vi "sub_EasyIsel.vi"(0 "x-Position":dbl, 1 "y-Position":dbl, 2 "z-Position":dbl, 3 "Velocity (x)":dbl=2000.0, 4 "Velocity (y)":dbl=500.0, 5 "Velocity (z)":dbl=4000.0, 6 "VISA resource name":refnum<visa-resource-name>="COM4", 8 "Mode":enum16{"Position", "Move", "Stop", "Home"}(ring), 9 "Steps/mm (y)":dbl=157.0, 11 "Steps/mm (z)":dbl=157.0) -> (14 "x-Position":dbl=6428.828025477707, 15 "y-Position":dbl, 16 "z-Position":dbl, 17 "Errorcode":string)   [LabVIEW 2014]
uses:
  <vilib>/Instr/_visa.llb/VISA Configure Serial Port (Instr).vi
panel:
  in  "Steps/mm (x)":dbl=157.0
  # "Set Steps/mm (x) to 157! (Markus)"
  # "Set Steps/mm (z) to 157! (Markus)"
  # "Description:\n\nFour different modes: Move, Position, Home, Stop\n\nMove: Move to position (absolute)\n\nPosition: Get position (x, y, z)\n\nHome: Set home\n\nStop: Stops movement and writes position (but resets controller -> new home)"
  # "Manuel Weiss, 13.08.2015"
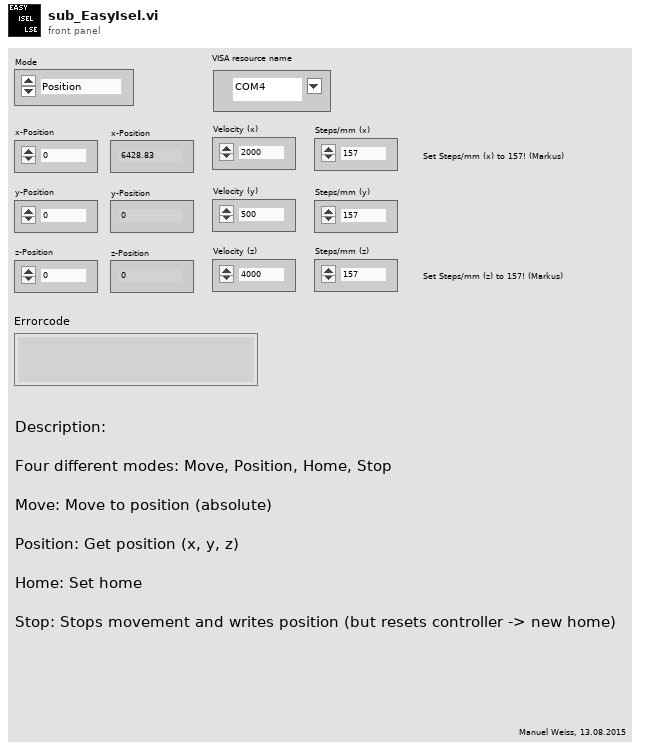
[diagram p1: front panel]
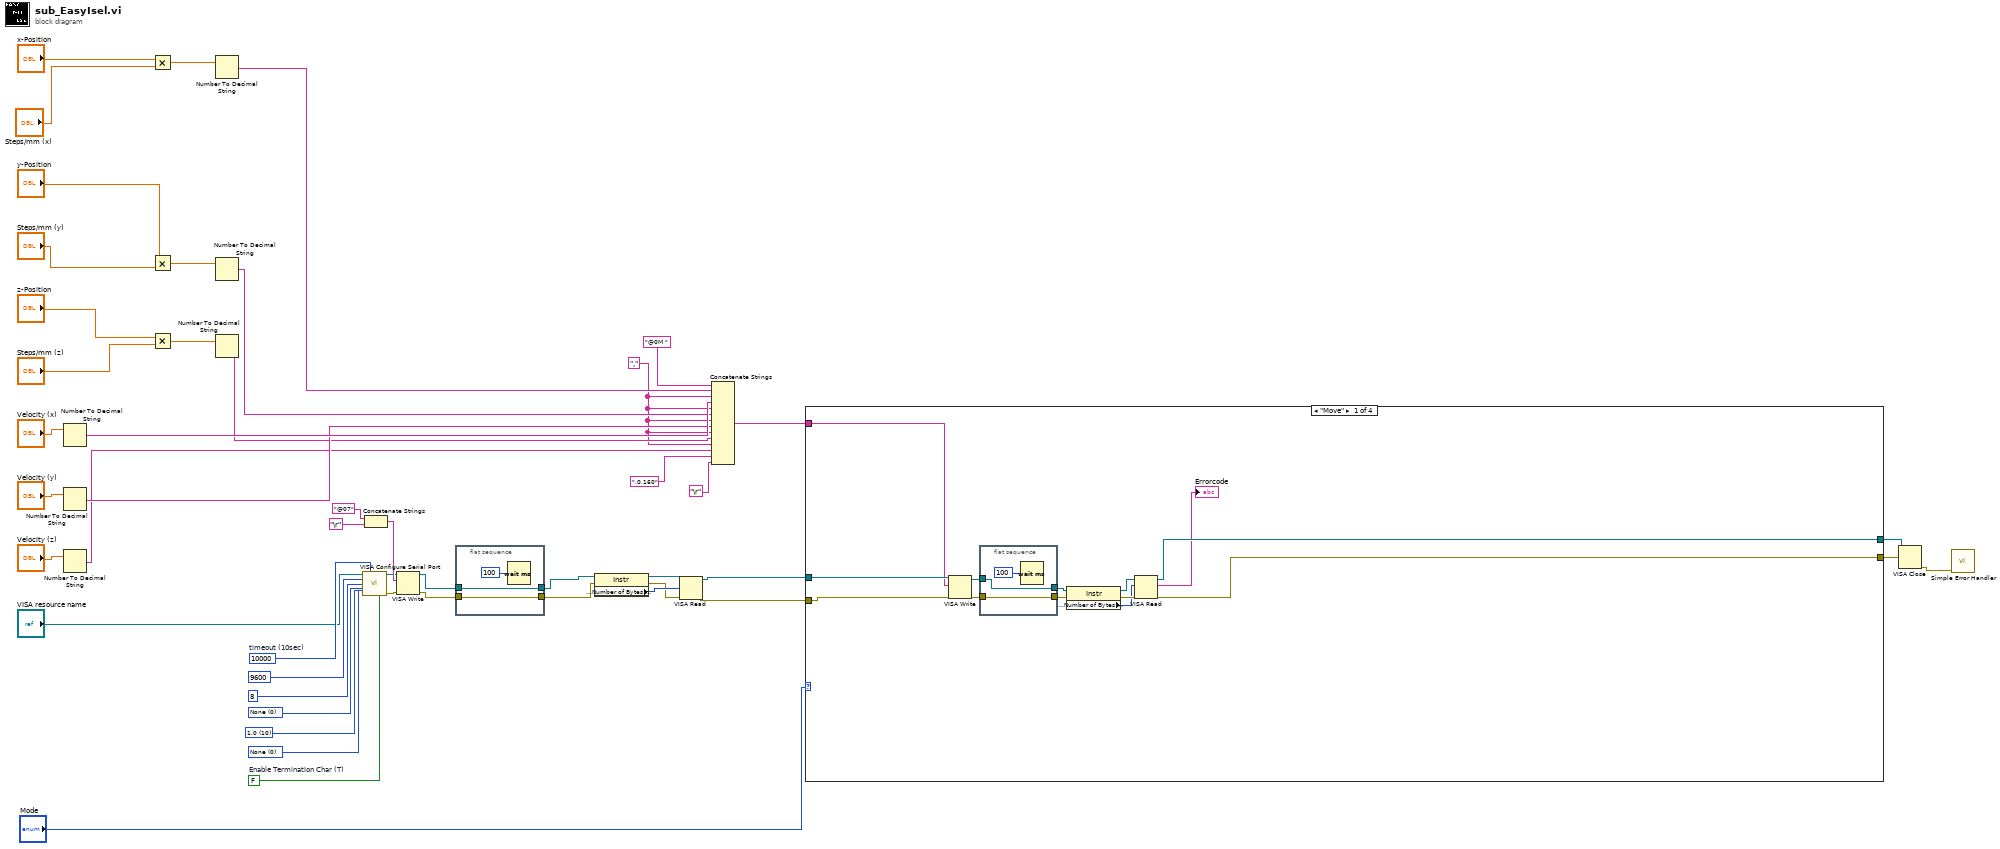
[diagram p0: block diagram]
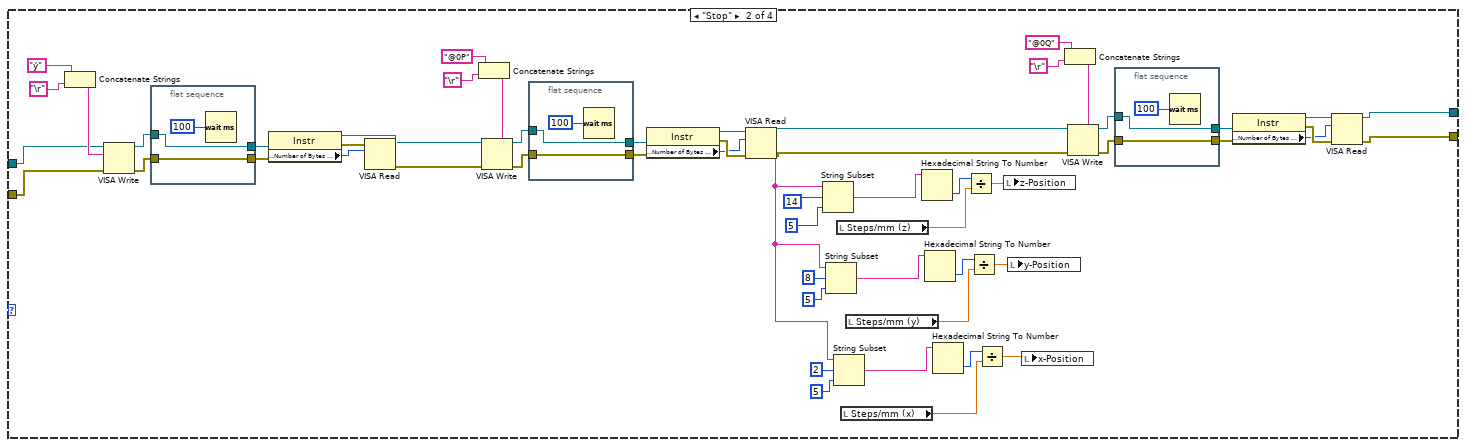
[diagram p2: hidden frame]
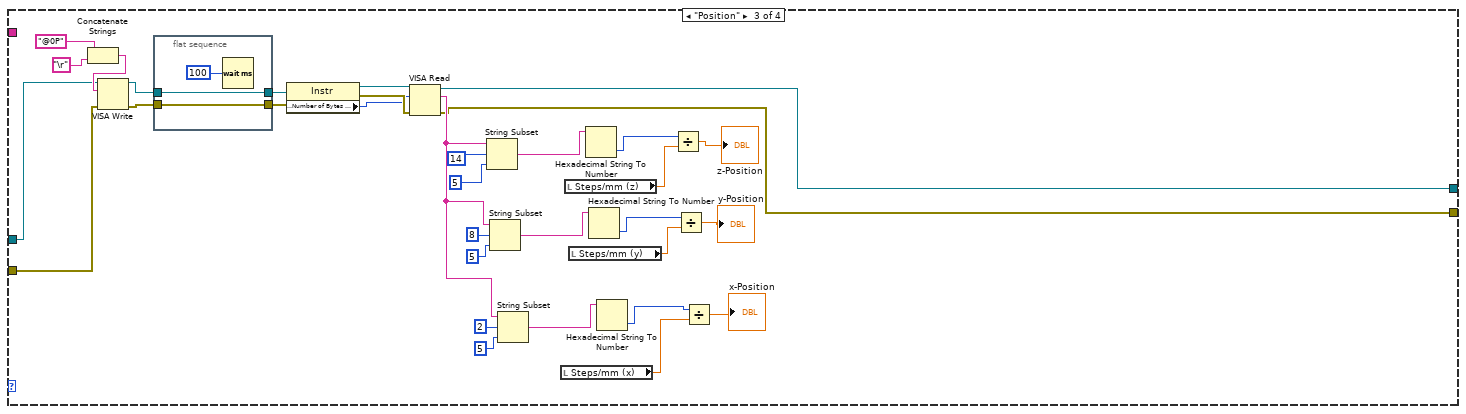
[diagram p3: hidden frame]
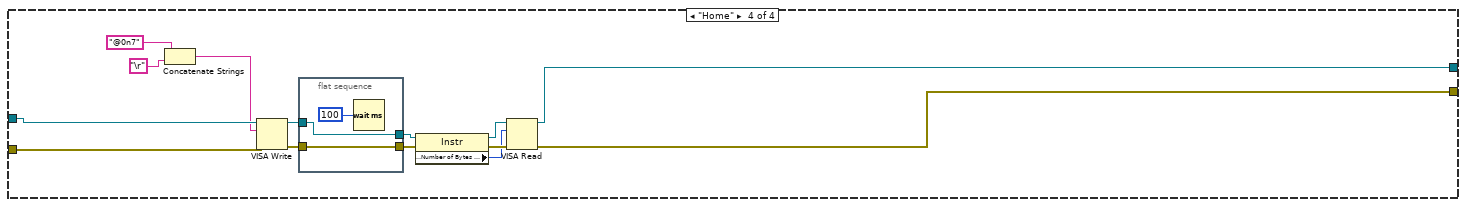
[diagram p4: hidden frame]
diagram:
  w22 = "," ("string")
  w45 = u16 0 items=["None"=0, "XON/XOFF"=1, "RTS/CTS"=2, "DTR/DSR"=4] ("flow control")
  w43 = u16 10 items=["1.0"=10, "1.5"=15, "2.0"=20] ("stop bits")
  w48 = u16 0 items=["None", "Odd", "Even", "Mark", "Space"] ("parity")
  w46 = FALSE  # Enable Termination Char (T)
  w47 = u32 10000  # timeout (10sec)
  n1 = Number To Decimal String(number="Velocity (x)") -> (decimal integer string=w26:string)  [unwired: 1 in]
  n2 = Number To Decimal String(number="Velocity (y)") -> (decimal integer string=w24:string)  [unwired: 1 in]
  n3 = Number To Decimal String(number="Velocity (z)") -> (decimal integer string=w21:string)  [unwired: 1 in]
  n4 = Multiply(x="x-Position", y="Steps/mm (x)") -> (x*y=w34:dbl)
  n5 = Multiply(x="y-Position", y="Steps/mm (y)") -> (x*y=w33:dbl)
  n6 = Multiply(x="z-Position", y="Steps/mm (z)") -> (x*y=w32:dbl)
  n7 = Number To Decimal String(number=w34) -> (decimal integer string=w27:string)  [unwired: 1 in]
  n8 = Number To Decimal String(number=w33) -> (decimal integer string=w25:string)  [unwired: 1 in]
  n9 = Number To Decimal String(number=w32) -> (decimal integer string=w23:string)  [unwired: 1 in]
  n10 = call-poly "VISA Configure Serial Port"("VISA resource name"="VISA resource name", "timeout (10sec)"=w47, "Enable Termination\nChar (T)"=w46, "baud rate (9600)"=u32 9600 ("baud rate"), "data bits (8)"=u16 8 ("data bits"), "parity (0:none)"=w48, "stop bits (10: 1 bit)"=w43, "flow control (0:none)"=w45) -> ("VISA resource name out"=w39:refnum<visa-resource-name>, "error out"=w38:errorcluster)  [unwired: 6 in]
  n11 = Concatenate Strings("@07" ("string"), "\r") -> (w40:string)
  n12 = VISA Write(VISA resource name=w39, write buffer=w40, error in (no error)=w38) -> (VISA resource name out=w15:refnum<visa-resource-name>, error out=w14:errorcluster)  [unwired: 1 out]
  n13 = flat-sequence {
    tunnel: w15 -> [w51]
    tunnel: [w52] -> w12
    tunnel: w14 -> [w52]
    tunnel: [w51] -> w13
    frame #0 {
      n14 = Wait (ms)(milliseconds to wait=u32 100) -> ()  [unwired: 1 out]
    }
  }
  n15 = property class="Instr"(reference=w13, error in=w12) -> (reference out=w18:refnum<visa-resource-name>, error out=w16:errorcluster, "Serial Settings:Number of Bytes at Serial Port"=w17:u32)
  n16 = VISA Read(VISA resource name=w18, byte count=w17, error in (no error)=w16) -> (VISA resource name out=w11:refnum<visa-resource-name>, error out=w10:errorcluster)  [unwired: 2 out]
  n17 = Concatenate Strings("@0M " ("string"), w27, w22, w26, w22, w25, w22, w24, w22, w23, w22, w21, ",0,160" ("string"), "\r") -> (w6:string)
  n18 = case shown="\"Move\"" "Mode" {
    tunnel: w11 -> [w58 w115 w140 w177]
    tunnel: w10 -> [w57 w114 w141 w176]
    tunnel: w6 -> [w56 _ _ _]
    tunnel: [w54 w77 w143 w174] -> w4
    tunnel: [w55 w78 w142 w175] -> w3
    frame "Move" {
      n19 = VISA Write(VISA resource name=w58, write buffer=w56, error in (no error)=w57) -> (VISA resource name out=w64:refnum<visa-resource-name>, error out=w62:errorcluster)  [unwired: 1 out]
      n20 = flat-sequence {
        tunnel: w64 -> [w67]
        tunnel: [w68] -> w63
        tunnel: w62 -> [w68]
        tunnel: [w67] -> w61
        frame #0 {
          n21 = Wait (ms)(milliseconds to wait=u32 100) -> ()  [unwired: 1 out]
        }
      }
      n22 = property class="Instr"(reference=w61, error in=w63) -> (reference out=w60:refnum<visa-resource-name>, error out=w65:errorcluster, "Serial Settings:Number of Bytes at Serial Port"=w59:u32)
      n23 = VISA Read(VISA resource name=w60, byte count=w59, error in (no error)=w65) -> (VISA resource name out=w54:refnum<visa-resource-name>, read buffer=→"Errorcode":string, error out=w55:errorcluster)  [unwired: 1 out]
    }
    frame "Stop" {
      n24 = Concatenate Strings("ý" ("write buffer"), "\r") -> (w116:string)
      n25 = VISA Write(VISA resource name=w115, write buffer=w116, error in (no error)=w114) -> (VISA resource name out=w124:refnum<visa-resource-name>, error out=w122:errorcluster)  [unwired: 1 out]
      n26 = flat-sequence {
        tunnel: w124 -> [w133]
        tunnel: [w134] -> w123
        tunnel: w122 -> [w134]
        tunnel: [w133] -> w121
        frame #0 {
          n27 = Wait (ms)(milliseconds to wait=u32 100) -> ()  [unwired: 1 out]
        }
      }
      n28 = property class="Instr"(reference=w121, error in=w123) -> (reference out=w120:refnum<visa-resource-name>, error out=w125:errorcluster, "Serial Settings:Number of Bytes at Serial Port"=w119:u32)
      n29 = VISA Read(VISA resource name=w120, byte count=w119, error in (no error)=w125) -> (VISA resource name out=w105:refnum<visa-resource-name>, error out=w106:errorcluster)  [unwired: 2 out]
      n30 = Concatenate Strings("@0P" ("write buffer"), "\r") -> (w107:string)
      n31 = VISA Write(VISA resource name=w105, write buffer=w107, error in (no error)=w106) -> (VISA resource name out=w113:refnum<visa-resource-name>, error out=w111:errorcluster)  [unwired: 1 out]
      n32 = flat-sequence {
        tunnel: w113 -> [w130]
        tunnel: [w131] -> w112
        tunnel: w111 -> [w131]
        tunnel: [w130] -> w110
        frame #0 {
          n33 = Wait (ms)(milliseconds to wait=u32 100) -> ()  [unwired: 1 out]
        }
      }
      n34 = property class="Instr"(reference=w110, error in=w112) -> (reference out=w94:refnum<visa-resource-name>, error out=w93:errorcluster, "Serial Settings:Number of Bytes at Serial Port"=w92:u32)
      n35 = VISA Read(VISA resource name=w94, byte count=w92, error in (no error)=w93) -> (VISA resource name out=w76:refnum<visa-resource-name>, read buffer=w95:string, error out=w75:errorcluster)  [unwired: 1 out]
      n36 = String Subset(string=w95, offset (0)=14, length (rest)=5 ("length (rest)")) -> (substring=w69:string)
      n37 = String Subset(string=w95, offset (0)=8, length (rest)=5 ("length (rest)")) -> (substring=w70:string)
      n38 = String Subset(string=w95, offset (0)=2, length (rest)=5 ("length (rest)")) -> (substring=w71:string)
      n39 = local read "Steps/mm (z)"() -> (w91:dbl)
      n40 = local read "Steps/mm (x)"() -> (w89:dbl)
      n41 = local read "Steps/mm (y)"() -> (w90:dbl)
      n42 = Hexadecimal String To Number(string=w69) -> (number=w102:u32)  [unwired: 2 in, 1 out]
      n43 = Hexadecimal String To Number(string=w70) -> (number=w100:u32)  [unwired: 2 in, 1 out]
      n44 = Hexadecimal String To Number(string=w71) -> (number=w98:u32)  [unwired: 2 in, 1 out]
      n45 = Divide(x=w102, y=w91) -> (x/y=w74:dbl)
      n46 = Divide(x=w100, y=w90) -> (x/y=w73:dbl)
      n47 = Divide(x=w98, y=w89) -> (x/y=w72:dbl)
      n48 = local write "z-Position"(w74) -> ()
      n49 = local write "y-Position"(w73) -> ()
      n50 = local write "x-Position"(w72) -> ()
      n51 = Concatenate Strings("@0Q" ("write buffer"), "\r") -> (w82:string)
      n52 = VISA Write(VISA resource name=w76, write buffer=w82, error in (no error)=w75) -> (VISA resource name out=w88:refnum<visa-resource-name>, error out=w86:errorcluster)  [unwired: 1 out]
      n53 = flat-sequence {
        tunnel: w88 -> [w127]
        tunnel: [w128] -> w87
        tunnel: w86 -> [w128]
        tunnel: [w127] -> w85
        frame #0 {
          n54 = Wait (ms)(milliseconds to wait=u32 100) -> ()  [unwired: 1 out]
        }
      }
      n55 = property class="Instr"(reference=w85, error in=w87) -> (reference out=w81:refnum<visa-resource-name>, error out=w80:errorcluster, "Serial Settings:Number of Bytes at Serial Port"=w79:u32)
      n56 = VISA Read(VISA resource name=w81, byte count=w79, error in (no error)=w80) -> (VISA resource name out=w77:refnum<visa-resource-name>, error out=w78:errorcluster)  [unwired: 2 out]
    }
    frame "Position" {
      n57 = Concatenate Strings("@0P" ("write buffer"), "\r") -> (w145:string)
      n58 = VISA Write(VISA resource name=w140, write buffer=w145, error in (no error)=w141) -> (VISA resource name out=w154:refnum<visa-resource-name>, error out=w153:errorcluster)  [unwired: 1 out]
      n59 = flat-sequence {
        tunnel: w154 -> [w169]
        tunnel: [w170] -> w151
        tunnel: w153 -> [w170]
        tunnel: [w169] -> w152
        frame #0 {
          n60 = Wait (ms)(milliseconds to wait=u32 100) -> ()  [unwired: 1 out]
        }
      }
      n61 = property class="Instr"(reference=w152, error in=w151) -> (reference out=w150:refnum<visa-resource-name>, error out=w149:errorcluster, "Serial Settings:Number of Bytes at Serial Port"=w147:u32)
      n62 = VISA Read(VISA resource name=w150, byte count=w147, error in (no error)=w149) -> (VISA resource name out=w143:refnum<visa-resource-name>, read buffer=w146:string, error out=w142:errorcluster)  [unwired: 1 out]
      n63 = String Subset(string=w146, offset (0)=14, length (rest)=5 ("length (rest)")) -> (substring=w165:string)
      n64 = String Subset(string=w146, offset (0)=8, length (rest)=5 ("length (rest)")) -> (substring=w161:string)
      n65 = String Subset(string=w146, offset (0)=2, length (rest)=5 ("length (rest)")) -> (substring=w158:string)
      n66 = local read "Steps/mm (x)"() -> (w157:dbl)
      n67 = local read "Steps/mm (z)"() -> (w164:dbl)
      n68 = local read "Steps/mm (y)"() -> (w160:dbl)
      n69 = Hexadecimal String To Number(string=w165) -> (number=w163:u32)  [unwired: 2 in, 1 out]
      n70 = Hexadecimal String To Number(string=w161) -> (number=w136:u32)  [unwired: 2 in, 1 out]
      n71 = Hexadecimal String To Number(string=w158) -> (number=w135:u32)  [unwired: 2 in, 1 out]
      n72 = Divide(x=w163, y=w164) -> (x/y=→"z-Position":dbl)
      n73 = Divide(x=w136, y=w160) -> (x/y=→"y-Position":dbl)
      n74 = Divide(x=w135, y=w157) -> (x/y=→"x-Position":dbl)
    }
    frame "Home" {
      n75 = Concatenate Strings("@0n7" ("write buffer"), "\r") -> (w171:string)
      n76 = VISA Write(VISA resource name=w177, write buffer=w171, error in (no error)=w176) -> (VISA resource name out=w183:refnum<visa-resource-name>, error out=w181:errorcluster)  [unwired: 1 out]
      n77 = flat-sequence {
        tunnel: w183 -> [w186]
        tunnel: [w187] -> w182
        tunnel: w181 -> [w187]
        tunnel: [w186] -> w180
        frame #0 {
          n78 = Wait (ms)(milliseconds to wait=u32 100) -> ()  [unwired: 1 out]
        }
      }
      n79 = property class="Instr"(reference=w180, error in=w182) -> (reference out=w179:refnum<visa-resource-name>, error out=w184:errorcluster, "Serial Settings:Number of Bytes at Serial Port"=w178:u32)
      n80 = VISA Read(VISA resource name=w179, byte count=w178, error in (no error)=w184) -> (VISA resource name out=w174:refnum<visa-resource-name>, error out=w175:errorcluster)  [unwired: 2 out]
    }
  }
  n81 = VISA Close(VISA resource name=w4, error in (no error)=w3) -> (error out=w5:errorcluster)
  n82 = call <vilib>:"Simple Error Handler.vi"("error in (no error)"=w5) -> ()  [unwired: 4 in, 5 out]
